vi "Validate Tree.vi"(11 "Branch Reference In":refnum<data-value>) -> (2 "error out":errorcluster, 3 "Branch Reference Out":refnum<data-value>)   [LabVIEW 2019, in "Tree.lvclass"]
uses:
  Tree.lvclass
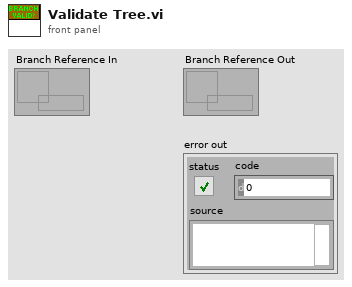
[diagram p1: front panel]
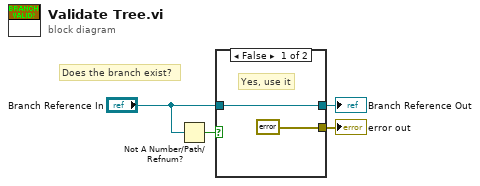
[diagram p0: block diagram]
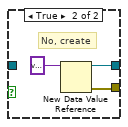
[diagram p2: hidden frame]
diagram:
  # "Does the branch exist?"
  n1 = Not A Number/Path/Refnum?(number/path/refnum="Branch Reference In") -> (NaN/Path/Refnum?=w4:bool)
  n2 = case shown="False" w4 {
    tunnel: "Branch Reference In" -> [w6 _]
    tunnel: [w6 w9] -> w2
    tunnel: [errorcluster {"status"=FALSE, "code"=0, "source"=""} ("error out") w7] -> w1
    frame False {
      # "Yes, use it"
    }
    frame True {
      # "No, create"
      n3 = New Data Value Reference(data value=variant) -> (data value reference=w9:refnum<data-value>, error out=w7:errorcluster)  [unwired: 1 in]
    }
  }
  "Branch Reference Out" <- w2
  "error out" <- w1
